vi "Obtain Status.vi"(8 "error in (no error)":errorcluster, 11 "Result in":refnum<class "Result.lvclass">) -> (0 "error out":errorcluster, 1 "String":string, 2 "Page":T1(ring), 3 "Result out":refnum<class "Result.lvclass">)   [LabVIEW 2023, in "Result.lvclass"]
uses:
  Result.lvclass
  Result.lvclass/Result.ctl
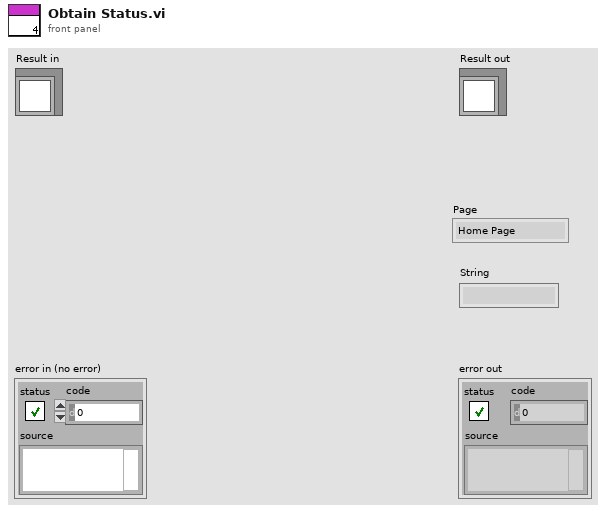
[diagram p1: front panel]
types:
  T1 = enum32{"Home Page", "Mode Page", "Configuration Page", "Input Page", "Result Page"}
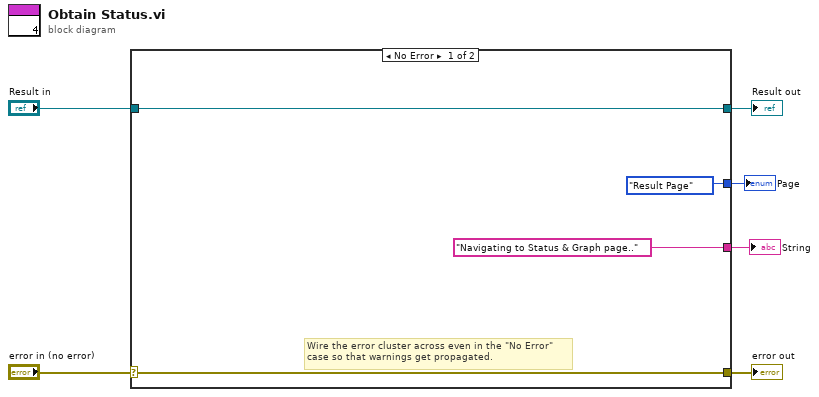
[diagram p0: block diagram]
diagram:
  n1 = case shown="No Error" "error in (no error)" {
    selector: "error in (no error)" -> [w9 w12]
    tunnel: [w9 w12] -> w5
    tunnel: [w10 w11] -> w3
    tunnel: "Result in" -> [w10 w11]
    tunnel: [T1."Result Page" ("Page") _] -> w2
    tunnel: ["Navigating to Status & Graph page.." ("String 2") _] -> w1
    frame No Error {
      # "Wire the error cluster across even in the \"No Error\"\ncase so that warnings get propagated."
    }
    frame Error {
    }
  }
  "error out" <- w5
  "Result out" <- w3
  "Page" <- w2
  "String" <- w1
